vi "GetPoint.vi"(8 "error in (no error)":errorcluster, 11 "Line in":refnum<class "Line.lvclass">) -> (0 "error out":errorcluster, 2 "Point":refnum<class "Point.lvclass">, 3 "Line out":refnum<class "Line.lvclass">)   [LabVIEW 2021, in "Picture2D.lvlib" / "Line.lvclass"]
uses:
  Line.lvclass
  Shape/Shape.lvclass
  Point/Point.lvclass
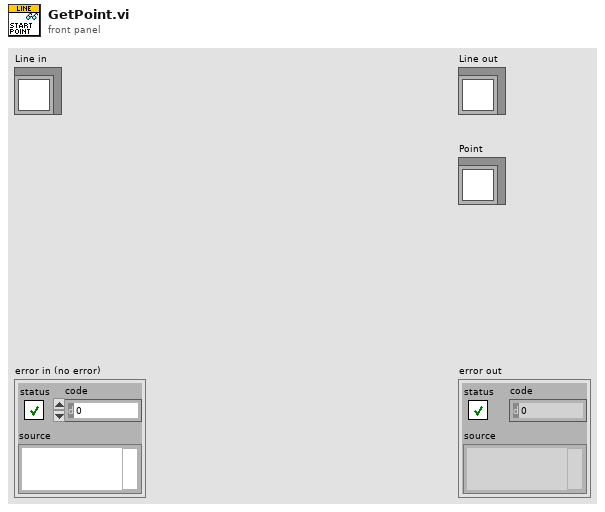
[diagram p1: front panel]
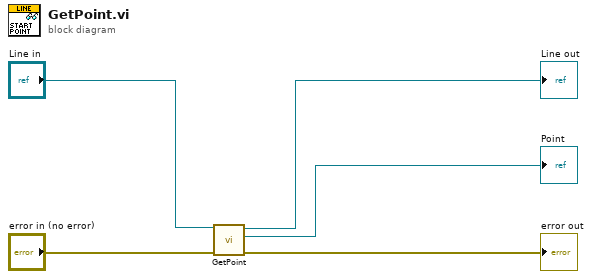
[diagram p0: block diagram]
diagram:
  n1 = call-parent "GetPoint.vi"("error in (no error)"="error in (no error)", "Picture2D in"="Line in") -> ("error out"=→"error out":errorcluster, "Point"=→"Point":refnum<class "Point.lvclass">, "Picture2D out"=→"Line out":refnum<class "Line.lvclass">)  [unwired: 7 in]
